vi "fgv_cpu-memory_usage.vi"(7 "cmd":enum16{"ini", "check", "close"}(ring), 8 "error in":errorcluster) -> (0 "error out":errorcluster, 2 "Mem. Usage":sgl format="%.2p", 3 "CPU Usage":sgl)   [LabVIEW 2019]
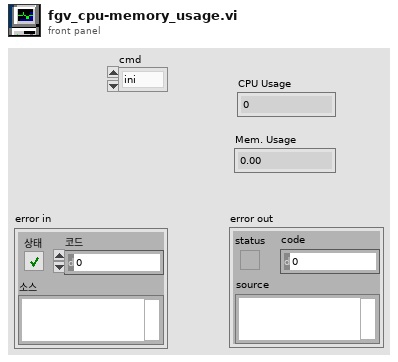
[diagram p1: front panel]
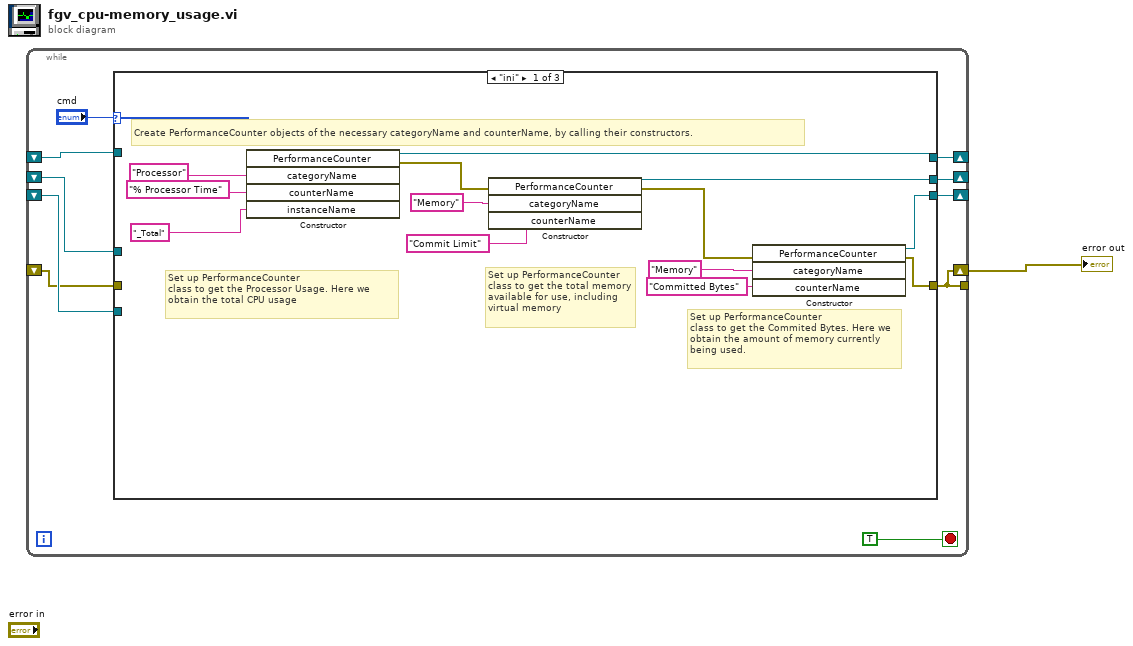
[diagram p0: block diagram]
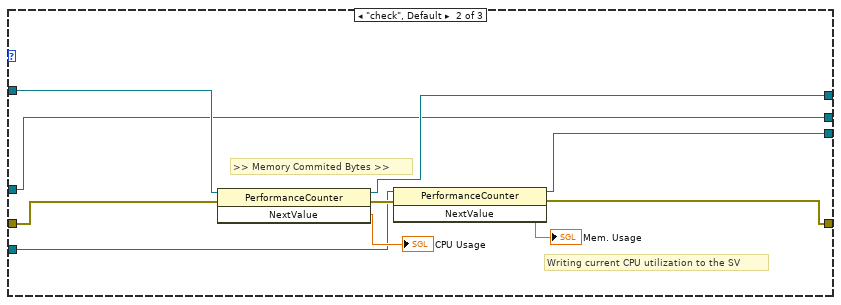
[diagram p2: hidden frame]
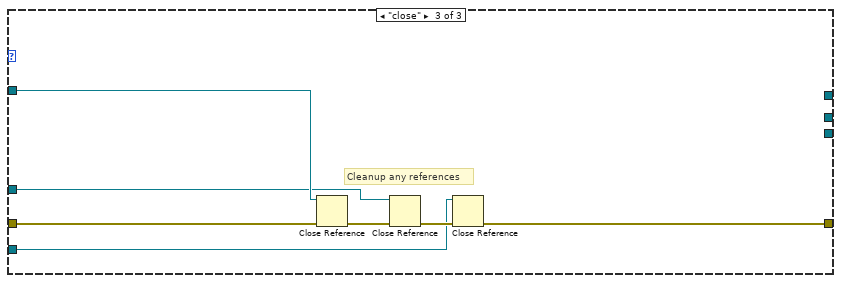
[diagram p3: hidden frame]
diagram:
  n1 = while {
    shift-right: [w7] -> _
    shift-left: _ -> [w6]
    shift-right: [w8] -> _
    shift-left: _ -> [w5]
    shift-right: [w9] -> _
    shift-left: _ -> [w4]
    shift-right: [w3] -> w1
    shift-left: _ -> [w2]
    tunnel: [w3] -> _
    stop <- TRUE stop-if-true
    n2 = case shown="\"ini\"" "cmd" {
      tunnel: [w18 w29 _] -> w9
      tunnel: [w17 w25 _] -> w8
      tunnel: [w16 w26 _] -> w7
      tunnel: w6 -> [_ w28 w39]
      tunnel: w5 -> [_ w25 w38]
      tunnel: w4 -> [_ w27 w37]
      tunnel: [w15 w30 w36] -> w3
      tunnel: w2 -> [_ w31 w35]
      frame "ini" {
        # "Create PerformanceCounter objects of the necessary categoryName and counterName, by calling their constructors."
        # "Set up PerformanceCounter \nclass to get the total memory available for use, including virtual memory"
        # "Set up PerformanceCounter \nclass to get the Commited Bytes. Here we obtain the amount of memory currently being used."
        # "Set up PerformanceCounter \nclass to get the Processor Usage. Here we obtain the total CPU usage"
        n3 = constructor class="PerformanceCounter"("categoryName"="Processor", "counterName"="% Processor Time", "instanceName"="_Total") -> (reference out=w16:refnum<k24>, error out=w20:errorcluster)  [unwired: 3 in, 4 out]
        n4 = constructor class="PerformanceCounter"(error in=w20, "categoryName"="Memory", "counterName"="Commit Limit") -> (reference out=w17:refnum<k24>, error out=w19:errorcluster)  [unwired: 2 in, 3 out]
        n5 = constructor class="PerformanceCounter"(error in=w19, "categoryName"="Memory", "counterName"="Committed Bytes") -> (reference out=w18:refnum<k24>, error out=w15:errorcluster)  [unwired: 2 in, 3 out]
      }
      frame "check", Default {
        # "Writing current CPU utilization to the SV"
        # ">> Memory Commited Bytes >>"
        n6 = invoke class="PerformanceCounter" method="NextValue"(reference=w28, error in=w31) -> (reference out=w26:refnum<k24>, error out=w34:errorcluster, "NextValue"=→"CPU Usage":sgl)  [unwired: 1 in]
        n7 = invoke class="PerformanceCounter" method="NextValue"(reference=w27, error in=w34) -> (reference out=w29:refnum<k24>, error out=w30:errorcluster, "NextValue"=→"Mem. Usage":sgl)  [unwired: 1 in]
      }
      frame "close" {
        # "Cleanup any references"
        n8 = Close Reference(reference=w39, error in (no error)=w35) -> (error out=w40:errorcluster)
        n9 = Close Reference(reference=w38, error in (no error)=w40) -> (error out=w41:errorcluster)
        n10 = Close Reference(reference=w37, error in (no error)=w41) -> (error out=w36:errorcluster)
      }
    }
  }
  "error out" <- w1
